vi "IECal-Options Dialog.vi"(0 "Override smoothing":T1={"Speaker"="", "Stimulus"={"Type"="", "Freq step (Hz)"=50.0, "Sampling rate (Hz)"=50000.0, "Attenuation (dB)"=20.0}, "Averages"=0, "Left gain"=0.0, "Right gain"=0.0, "plot max"=FALSE, "Max Vmic"=0.0}, 2 "Parent VI":refnum<vi>) -> (4 "Override Out":T1={"Speaker"="", "Stimulus"={"Type"="", "Freq step (Hz)"=50.0, "Sampling rate (Hz)"=50000.0, "Attenuation (dB)"=20.0}, "Averages"=0, "Left gain"=0.0, "Right gain"=0.0, "plot max"=FALSE, "Max Vmic"=0.0}, 8 "Canceled?":bool)   [LabVIEW 2020]
uses:
  Typedefs/IECal-Parameters.ctl
  Common VIs/Typedefs/CAL-Stimulus.ctl
panel:
  in  "Max Vmic":dbl caption="Maximum mic voltage" min=0.0 max=10.0
  in  "Cancel":bool
  in  "OK":bool
  # "In-Ear Calibration Options"
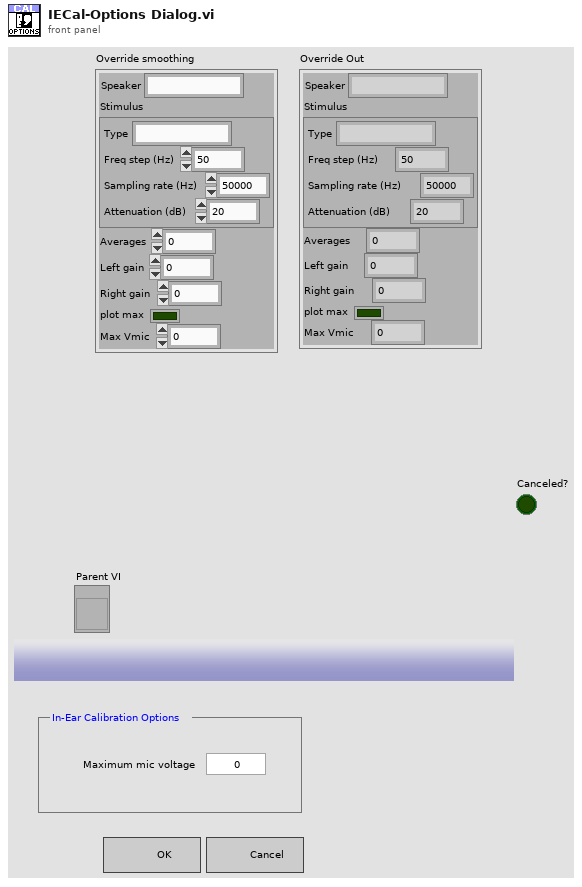
[diagram p1: front panel]
types:
  T1 = typedef "IECal-Parameters.ctl" = cluster{"Speaker":string, "Stimulus":T2, "Averages":i32, "Left gain":dbl, "Right gain":dbl, "plot max":bool, "Max Vmic":dbl}
  T2 = typedef "CAL-Stimulus.ctl" = cluster{"Type":string, "Freq step (Hz)":dbl, "Sampling rate (Hz)":dbl, "Attenuation (dB)":dbl}
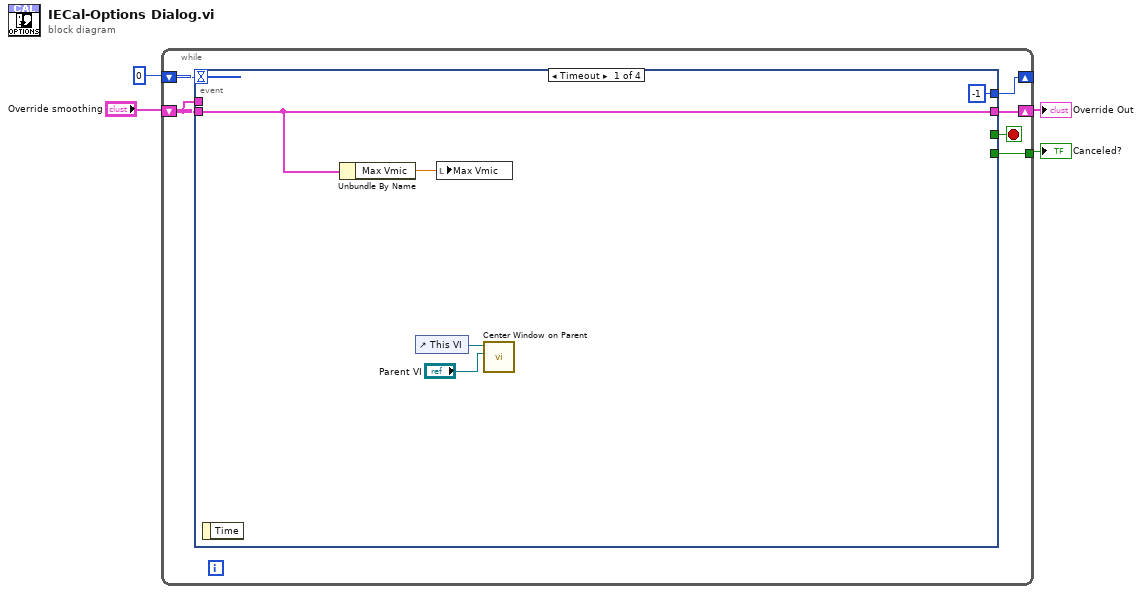
[diagram p0: block diagram]
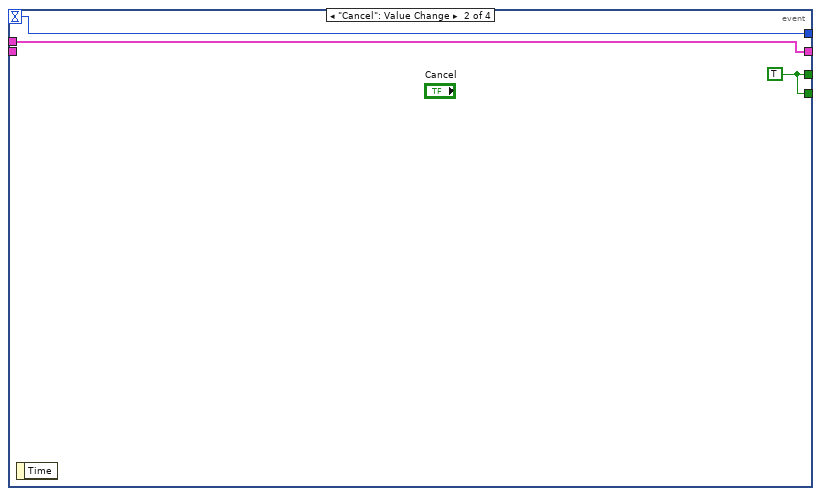
[diagram p2: hidden frame]
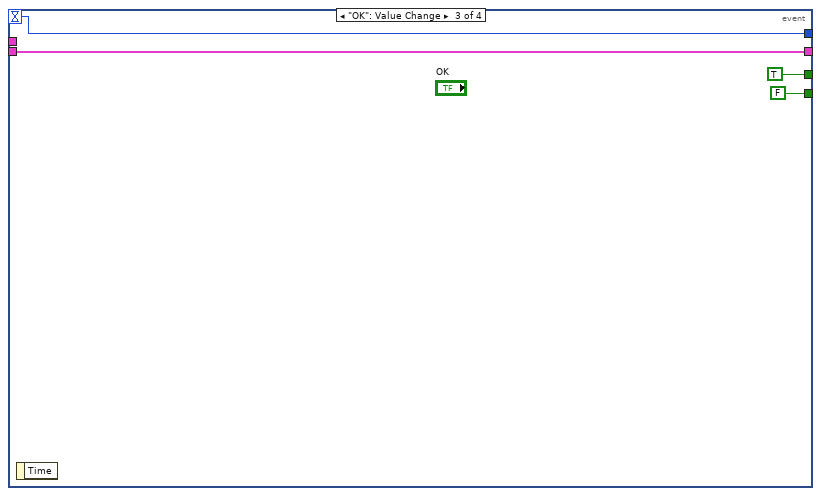
[diagram p3: hidden frame]
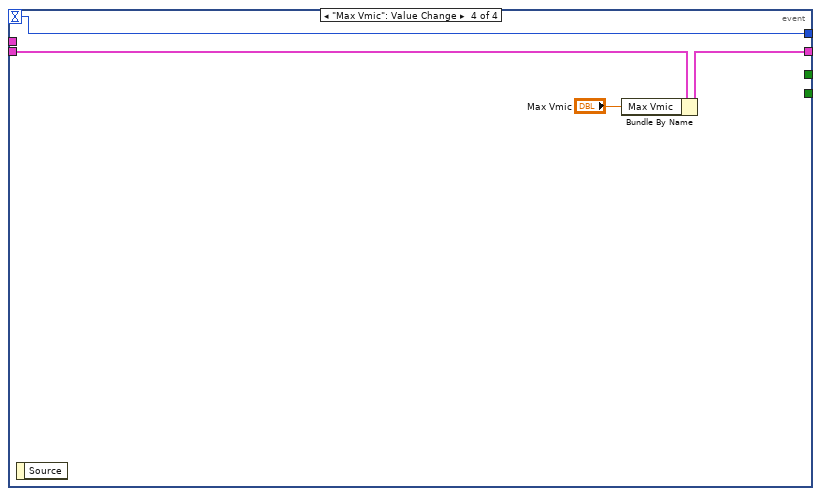
[diagram p4: hidden frame]
diagram:
  n1 = while {
    shift-right: [w9] -> _
    shift-left: 0 -> [w10]
    tunnel: [w6] -> w1
    shift-right: [w8] -> w2
    shift-left: "Override smoothing" -> [w5]
    stop <- w7 stop-if-true
    n2 = event shown="[0] Timeout" {
      selector: _ -> [_ _ _ _]
      dyn-events: _ -> [_ _ _ _]
      timeout: w10 -> [_ w18 w21 w26]
      tunnel: [-1 w18 w21 w26] -> w9
      tunnel: w5 -> [w14 _ w22 w25]
      tunnel: [w14 w16 w22 w24] -> w8
      tunnel: [_ w17 TRUE _] -> w7
      tunnel: [_ w17 FALSE _] -> w6
      tunnel: w5 -> [_ w16 _ _]
      event Timeout {
        n3 = event-data() -> ()  [unwired: 1 in, 1 out]
        n4 = Unbundle By Name(w14) -> ("Max Vmic"=w13:dbl)
        n5 = control-ref of="This VI"() -> (w12:refnum<vi>)
        n6 = local write "Max Vmic"(w13) -> ()
        n7 = call "Center Window on Parent.vi"("Parent VI"="Parent VI", "VI in"=w12) -> ()  [unwired: 8 in, 2 out]
      }
      event "Cancel": Value Change {
        w17 = TRUE
        n8 = event-data() -> ()  [unwired: 1 in, 1 out]
      }
      event "OK": Value Change {
        n9 = event-data() -> ()  [unwired: 1 in, 1 out]
      }
      event "Max Vmic": Value Change {
        n10 = event-data() -> ()  [unwired: 1 in, 1 out]
        n11 = Bundle By Name(cluster=w25, "Max Vmic"="Max Vmic") -> (w24:T1)
      }
    }
  }
  "Override Out" <- w2
  "Canceled?" <- w1
